vi "FindLast.vi"(8 "default":path, 9 "Task":enum16{"Save", "Read"}(ring), 11 "Tree":string) -> (2 "path":path)   [LabVIEW 2022 SP3]
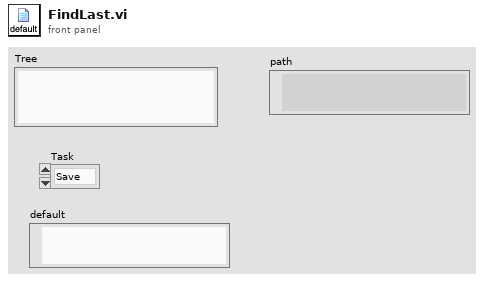
[diagram p1: front panel]
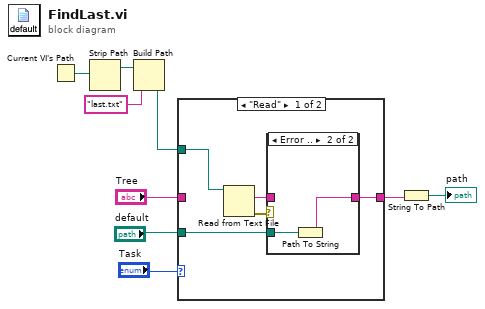
[diagram p0: block diagram]
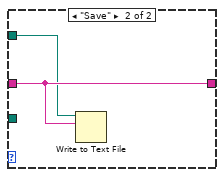
[diagram p3: hidden frame]
diagram:
  n1 = Current VI's Path() -> (path=w5:path)
  n2 = Strip Path(path=w5) -> (stripped path=w4:path)  [unwired: 1 out]
  n3 = Build Path(base path=w4, name or relative path="last.txt") -> (appended path=w3:path)
  n4 = case shown="\"Read\"" "Task" {
    tunnel: "Tree" -> [_ w19]
    tunnel: [w12 w19] -> w7
    tunnel: w3 -> [w14 w18]
    tunnel: "default" -> [w10 _]
    frame "Read" {
      n5 = Read from Text File(file (use dialog)=w14) -> (text=w11:string, error out=w13:errorcluster)  [unwired: 3 in, 2 out]
      n6 = case shown="Error .." w13 {
        tunnel: [w15 w16] -> w12
        tunnel: w11 -> [w15 _]
        tunnel: w10 -> [_ w17]
        frame No Error {
        }
        frame Error {
          n7 = Path To String(path=w17) -> (string=w16:string)
        }
      }
    }
    frame "Save" {
      n8 = Write to Text File(file (use dialog)=w18, text=w19) -> ()  [unwired: 2 in, 3 out]
    }
  }
  n9 = String To Path(string=w7) -> (path=→"path":path)
